vi "Convert_Always_Show_Info.vi"(7 "Raw Data (ERD Input)":T2[](array[typedef]) {"ERD Number" format="%.0x"}, 9 "ERD Headers":string[](array[string]), 11 "Error In":errorcluster, 12 "Enable Diagnostic Data":T1) -> (4 "Data":string[][](array[string]), 15 "Error Out":errorcluster)   [LabVIEW 2016, in "GEA2_Toolkit.lvlib"]
doc: "This VI parses the data from ERDs in correct format, units, etc. It handles all hex to dec conversions, hex to enum, and hex to boolean conversions.\n\nIf Raw Data from ERD is blank string, then it will output values from shift register."
uses:
  library/GEA2_Toolkit.lvlib
  type defs/ERD Read Data Out.ctl
  Washer HCC/Washer HCC NEWFI/Type Definitions/HCC Washer Types.ctl
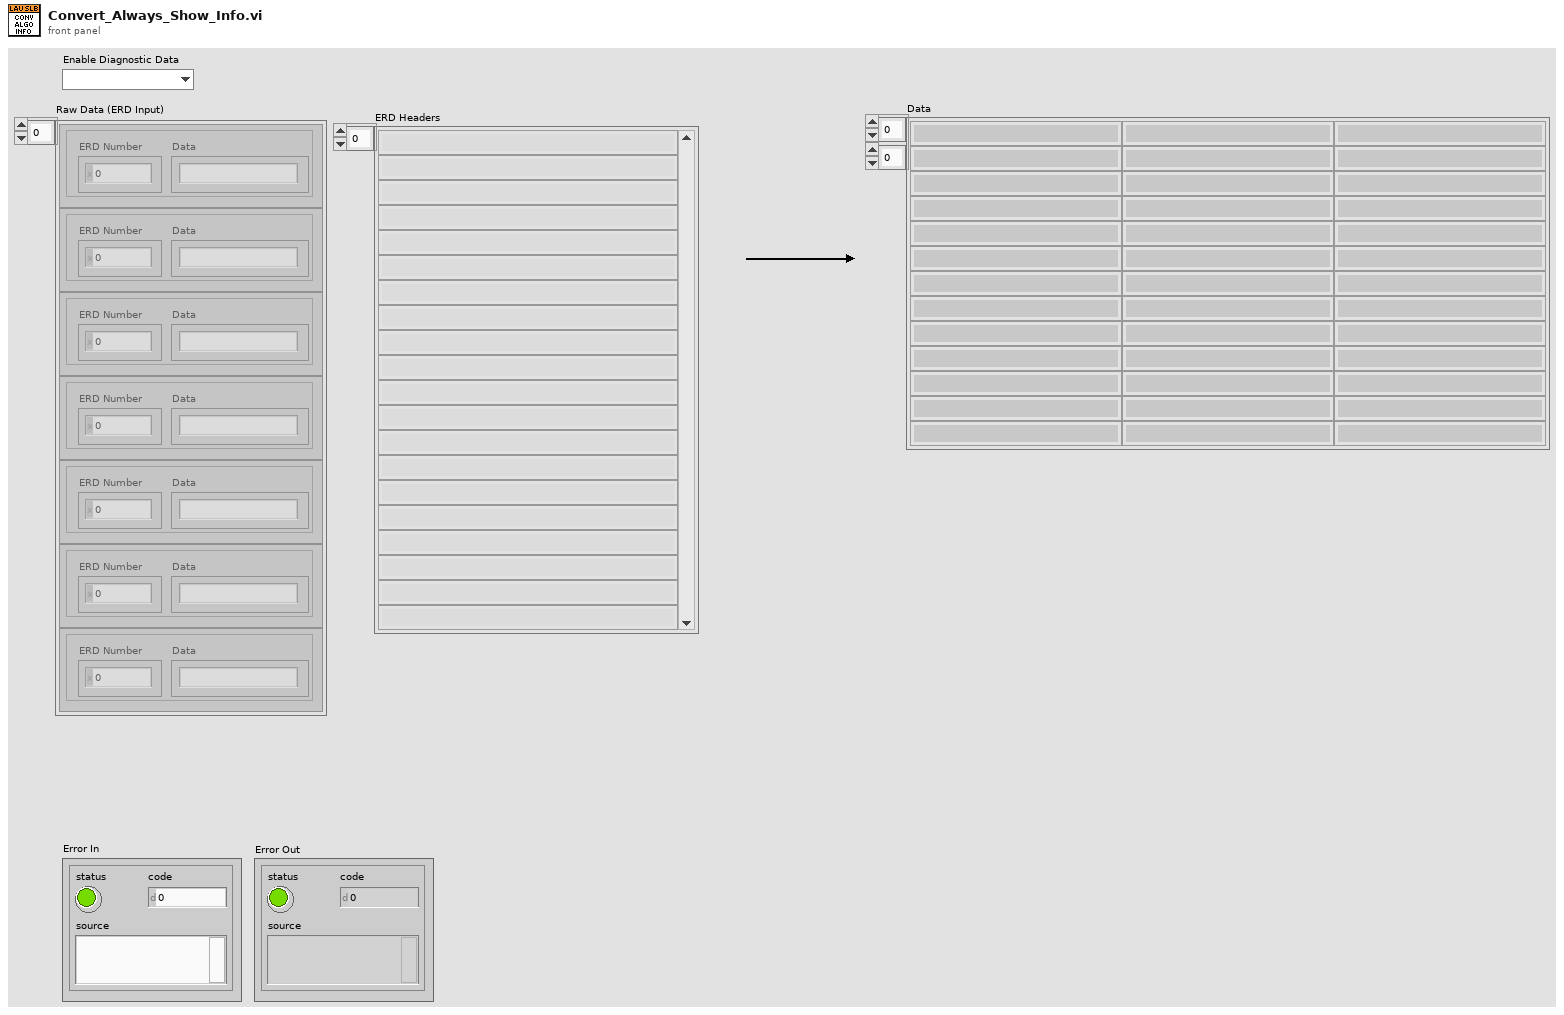
[diagram p1: front panel]
types:
  T1 = typedef "HCC Washer Types.ctl" = enum16{"", "Viper Washer", "Hawk Washer", "2015 Washer", "2017 Washer"}
  T2 = typedef "GEA2_Toolkit.lvlib/ERD Read Data Out.ctl" = cluster{"ERD Number":u16, "Data":string}
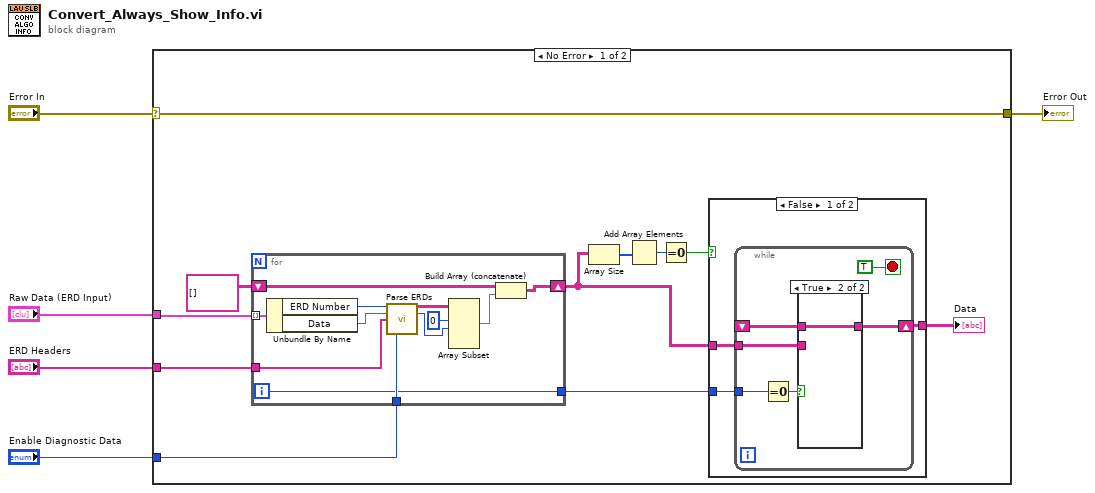
[diagram p0: block diagram]
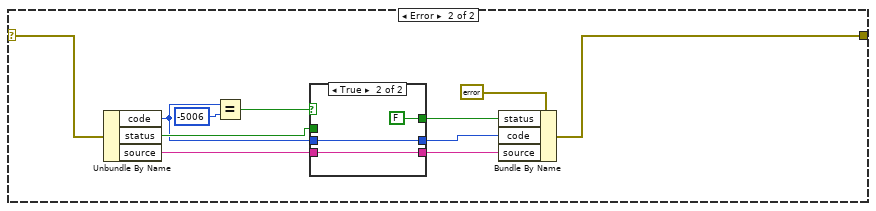
[diagram p4: hidden frame]
diagram:
  n1 = case shown="No Error" "Error In" {
    selector: "Error In" -> [w15 w42]
    tunnel: "Raw Data (ERD Input)" -> [w16 _]
    tunnel: [w15 w41] -> w3
    tunnel: "Enable Diagnostic Data" -> [w13 _]
    tunnel: "ERD Headers" -> [w10 _]
    frame No Error {
      n2 = for {
        tunnel: w16 -> [w40] mode=indexing
        shift-right: [w36] -> w9
        shift-left: string[][] [] -> [w37]
        tunnel: w13 -> [w31]
        tunnel: [w30] -> w12
        tunnel: w10 -> [w29]
        i -> [w30]
        n3 = Unbundle By Name(w40) -> ("ERD Number"=w39:u16, "Data"=w38:string)
        n4 = call "Parse ERDs.vi"("ERD Number"=w39, "Data"=w38, "ERD Headers"=w29, "Enable Diagnostic Data"=w31) -> ("Data"=w35:string[][], "Length"=w33:i32)  [unwired: 9 in, 1 out]
        n5 = Array Subset(array=w35, index (row)=0 ("index"), length (row)=w33) -> (w32:string[][])  [unwired: 2 in]
        n6 = Build Array (concatenate)(w37, w32) -> (w36:string[][])
      }
      n7 = Array Size(array=w9) -> (size(s)=w8:i32[])
      n8 = Add Array Elements(numeric array=w8) -> (sum=w7:i32)
      n9 = Equal To 0?(x=w7) -> (x = 0?=w6:bool)
      n10 = case shown="False" w6 {
        tunnel: w12 -> [w19 _]
        tunnel: [w18 w28] -> w11
        tunnel: w9 -> [w17 w28]
        frame False {
          n11 = while {
            shift-right: [w22] -> w18
            shift-left: _ -> [w21]
            tunnel: w19 -> [w25]
            tunnel: w17 -> [w23]
            stop <- TRUE stop-if-true
            n12 = Equal To 0?(x=w25) -> (x = 0?=w24:bool)
            n13 = case shown="True" w24 {
              tunnel: w23 -> [w26 _]
              tunnel: [w26 w27] -> w22
              tunnel: w21 -> [_ w27]
              frame False {
              }
              frame True {
              }
            }
          }
        }
        frame True {
        }
      }
      "Data" <- w11
    }
    frame Error {
      n14 = Unbundle By Name(w42) -> ("code"=w46:i32, "status"=w47:bool, "source"=w44:string)
      n15 = Equal?(x=w46, y=-5006) -> (x = y?=w50:bool)
      n16 = case shown="True" w50 {
        tunnel: [w54 FALSE] -> w48
        tunnel: w47 -> [w54 _]
        tunnel: w46 -> [w53 w56]
        tunnel: [w53 w56] -> w45
        tunnel: [w52 w55] -> w43
        tunnel: w44 -> [w52 w55]
        frame False {
        }
        frame True {
        }
      }
      n17 = Bundle By Name(cluster=errorcluster {"status"=FALSE, "code"=0, "source"=""} ("error constant"), "status"=w48, "code"=w45, "source"=w43) -> (w41:errorcluster)
    }
  }
  "Error Out" <- w3
